vi "InstrumentStudio styled controls.vi"() -> ()   [LabVIEW 2021]
panel:
  in  "output type":enum32{"Option 1", "Option 2", "Option 3"}(ring) caption="enum"
  in  "Settings 2":bool
  out "Error":bool
  in  "Settings":bool
  in  "Info":bool
  in  "Remove":bool
  in  "Move Up":bool
  in  "Move Down":bool
  in  "Add":bool
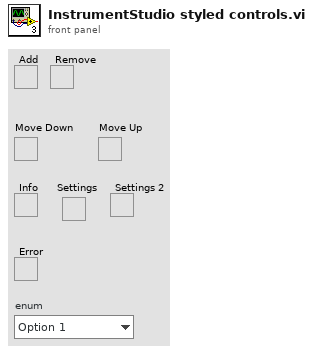
[diagram p1: front panel]
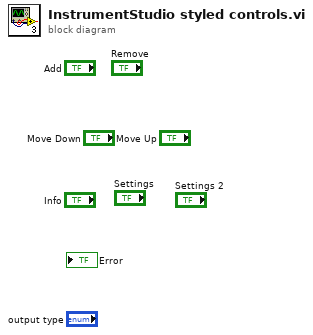
[diagram p0: block diagram]
diagram:
